vi "main.vi"() -> ()   [LabVIEW 2017]
uses:
  <vilib>/Instr/_visa.llb/VISA Configure Serial Port (Instr).vi
panel:
  in  "选项卡控件":enum32{"设置", "汽车状态", "电池状态", "单体电压", "单体温度"}(tab)
  in  "波特率":u32=19200
  in  "数据位":u16=8
  in  "奇偶位":enum16{"None", "Odd", "Even", "Mark", "Space"}(ring)
  in  "停止":bool
  in  "串口选择":refnum<visa-resource-name>="COM21"
  out "ID":string
  out "数据0":string
  out "数据1":string
  out "数据2":string
  out "数据3":string
  out "数据4":string
  out "数据5":string
  out "数据6":string
  out "数据7":string
  out "current time":timestamp
  out "error out":errorcluster
  out "轮速":u32(graph)
  out "单体温度断线告警":bool
  out "单体电压断线告警":bool
  out "充电状态":u8(ring) items=["停止充电", "进入充电", "恒流充电", "涓流充电", "充电完成"]
  out "车载充电器连接电阻":u8(ring) items=["InftyOmh", "220Omh", "680Omh", "未知电阻"]
  out "动力电池告警":bool
  out "动力电池告警级别":u32(ring) items=["无告警", "严重", "一般", "不严重"]
  out "动力电池总电压":dbl(graph)
  out "动力电池总电流":dbl(graph)
  out "剩余电量百分比":u32(graph)
  out "当前容量与出厂容量百分比":u32(graph)
  out "通信生命周期":u32(graph)
  out "动力电池状态":u32(ring) items=["无", "休眠", "自检", "待机", "预充", "正常运行", "关机", "故障"]
  out "最大允许充电功率":dbl
  out "最大允许充电电流":u16
  out "最大允许放电电流":u16
  out "最大允许放电功率":dbl
  out "加热控制":bool
  out "冷却控制":bool
  out "输出高压命令":bool
  out "关机命令":bool
  out "车载充电继电器开关":bool
  out "预充继电器开关":bool
  out "总负继电器开关":bool
  out "总正继电器开关":bool
  out "非车载充电继电器开关":bool
  out "非车载充电器连接确认":bool
  out "充电机在线":bool
  out "车载充电继电器错误":bool
  out "预充继电器错误":bool
  out "总负继电器错误":bool
  out "总正继电器错误":bool
  out "非车载充电继电器错误":bool
  out "车载充电器连接确认":bool
  out "充电请求电压":u16
  out "充电请求电流":u16
  out "电池低温告警级别":u8(ring) items=["无告警", "严重", "一般", "不严重"]
  out "电池低温告警":bool
  out "电池高温告警级别":u8(ring) items=["无告警", "严重", "一般", "不严重"]
  out "单体欠压告警":bool
  out "单体欠压告警级别":u8(ring) items=["无告警", "严重", "一般", "不严重"]
  out "单体过压告警":bool
  out "单体过压告警级别":u8(ring) items=["无告警", "严重", "一般", "不严重"]
  out "电池高温告警":bool
  out "稳态充电过流告警":bool
  out "电池组剩余电量百分比过低告警":bool caption="电池组剩余电量百分比过低告"
  out "电池组剩余电量百分比过高告警":bool
  out "整组欠压告警":bool
  out "被动均衡采集模块离线告警":bool
  out "整组过压告警":bool
  out "电池温差过大告警":bool
  out "电池压差过大告警":bool
  out "电池压差过大告警级别":u8(ring) items=["无告警", "严重", "一般", "不严重"]
  out "电池温差过大告警级别":u8(ring) items=["无告警", "严重", "一般", "不严重"]
  out "整组过压告警级别":u8(ring) items=["无告警", "严重", "一般", "不严重"]
  out "电池管理模块故障告警":bool
  out "继电器故障告警":bool
  out "预充失败告警":bool
  out "被动均衡采集模块均衡故障告警":bool
  out "霍尔断线告警":bool
  out "电池高压异常告警":bool
  out "漏电流超限告警级别":u8(ring) items=["无告警", "严重", "一般", "不严重"]
  out "漏电流超限告警":bool
  out "稳态放电过流告警级别":u8(ring) items=["无告警", "严重", "一般", "不严重"]
  out "稳态放电过流告警":bool
  out "整组欠压告警级别":u8(ring) items=["无告警", "严重", "一般", "不严重"]
  out "稳态充电过流告警级别":u8(ring) items=["无告警", "严重", "一般", "不严重"]
  out "瞬态充电过流告警":bool
  out "瞬态充电过流告警级别":u8(ring) items=["无告警", "严重", "一般", "不严重"]
  out "瞬态放电过流告警级别":u8(ring) items=["无告警", "严重", "一般", "不严重"]
  out "瞬态放电过流告警":bool
  out "电池组剩余电量百分比过低告警级别":u8(ring) items=["无告警", "严重", "一般", "不严重"]
  out "电池组剩余电量百分比过高告警级别":u8(ring) items=["无告警", "严重", "一般", "不严重"]
  out "整车控制模块通讯超时告警级别":u8(ring) items=["无告警", "严重", "一般", "不严重"]
  out "整车控制模块通讯超时告警":bool
  out "被动均衡采集模块离线告警级别":u8(ring) items=["无告警", "严重", "一般", "不严重"]
  in  "选项卡控件 2":T1(tab)
  out "最高单体电压":u16(graph)
  out "最低单体电压":u16(graph)
  out "最高单体电压序号":u32(graph)
  out "最低单体电压序号":u32(graph)
  out "单体电压2":u32(graph)
  out "单体电压5":u32(graph)
  out "单体电压6":u32(graph)
  out "单体电压7":u32(graph)
  out "单体电压0":u32(graph)
  out "单体电压1":u32(graph)
  out "单体电压3":u32(graph)
  out "单体电压4":u32(graph)
  out "单体电压10":u32(graph)
  out "单体电压13":u32(graph)
  out "单体电压14":u32(graph)
  out "单体电压15":u32(graph)
  out "单体电压8":u32(graph)
  out "单体电压9":u32(graph)
  out "单体电压11":u32(graph)
  out "单体电压12":u32(graph)
  out "单体电压21":u32(graph)
  out "单体电压18":u32(graph)
  out "单体电压23":u32(graph)
  out "单体电压17":u32(graph)
  out "单体电压20":u32(graph)
  out "单体电压22":u32(graph)
  out "单体电压16":u32(graph)
  out "单体电压19":u32(graph)
  out "单体电压30":u32(graph)
  out "单体电压28":u32(graph)
  out "单体电压25":u32(graph)
  out "单体电压31":u32(graph)
  out "单体电压26":u32(graph)
  out "单体电压29":u32(graph)
  out "单体电压24":u32(graph)
  out "单体电压27":u32(graph)
  out "单体电压38":u32(graph)
  out "单体电压36":u32(graph)
  out "单体电压33":u32(graph)
  out "单体电压39":u32(graph)
  out "单体电压34":u32(graph)
  out "单体电压37":u32(graph)
  out "单体电压32":u32(graph)
  out "单体电压35":u32(graph)
  out "单体电压46":u32(graph)
  out "单体电压44":u32(graph)
  out "单体电压41":u32(graph)
  out "单体电压47":u32(graph)
  out "单体电压42":u32(graph)
  out "单体电压45":u32(graph)
  out "单体电压40":u32(graph)
  out "单体电压43":u32(graph)
  in  "选项卡控件 3":T2(tab)
  out "最低温度序号":u32(graph)
  out "最低温度":u32(graph)
  out "最高温度":u32(graph)
  out "最高温度序号":u32(graph)
  out "单体温度0":u32(graph)
  out "单体温度1":u32(graph)
  out "单体温度2":u32(graph)
  out "单体温度3":u32(graph)
  out "单体温度4":u32(graph)
  out "单体温度6":u32(graph)
  out "单体温度7":u32(graph)
  out "单体温度5":u32(graph)
  out "单体温度8":u32(graph)
  out "单体温度9":u32(graph)
  out "单体温度10":u32(graph)
  out "单体温度11":u32(graph)
  out "单体温度12":u32(graph)
  out "单体温度14":u32(graph)
  out "单体温度15":u32(graph)
  out "单体温度13":u32(graph)
  out "单体温度16":u32(graph)
  out "单体温度17":u32(graph)
  out "单体温度18":u32(graph)
  out "单体温度19":u32(graph)
  out "单体温度20":u32(graph)
  out "单体温度22":u32(graph)
  out "单体温度23":u32(graph)
  out "单体温度21":u32(graph)
  out "单体温度29":u32(graph)
  out "单体温度31":u32(graph)
  out "单体温度30":u32(graph)
  out "单体温度28":u32(graph)
  out "单体温度27":u32(graph)
  out "单体温度26":u32(graph)
  out "单体温度25":u32(graph)
  out "单体温度24":u32(graph)
  out "单体温度32":u32(graph)
  out "单体温度33":u32(graph)
  out "单体温度34":u32(graph)
  out "单体温度35":u32(graph)
  out "单体温度36":u32(graph)
  out "单体温度38":u32(graph)
  out "单体温度39":u32(graph)
  out "单体温度37":u32(graph)
  out "单体温度40":u32(graph)
  out "单体温度41":u32(graph)
  out "单体温度42":u32(graph)
  out "单体温度43":u32(graph)
  out "单体温度44":u32(graph)
  out "单体温度46":u32(graph)
  out "单体温度47":u32(graph)
  out "单体温度45":u32(graph)
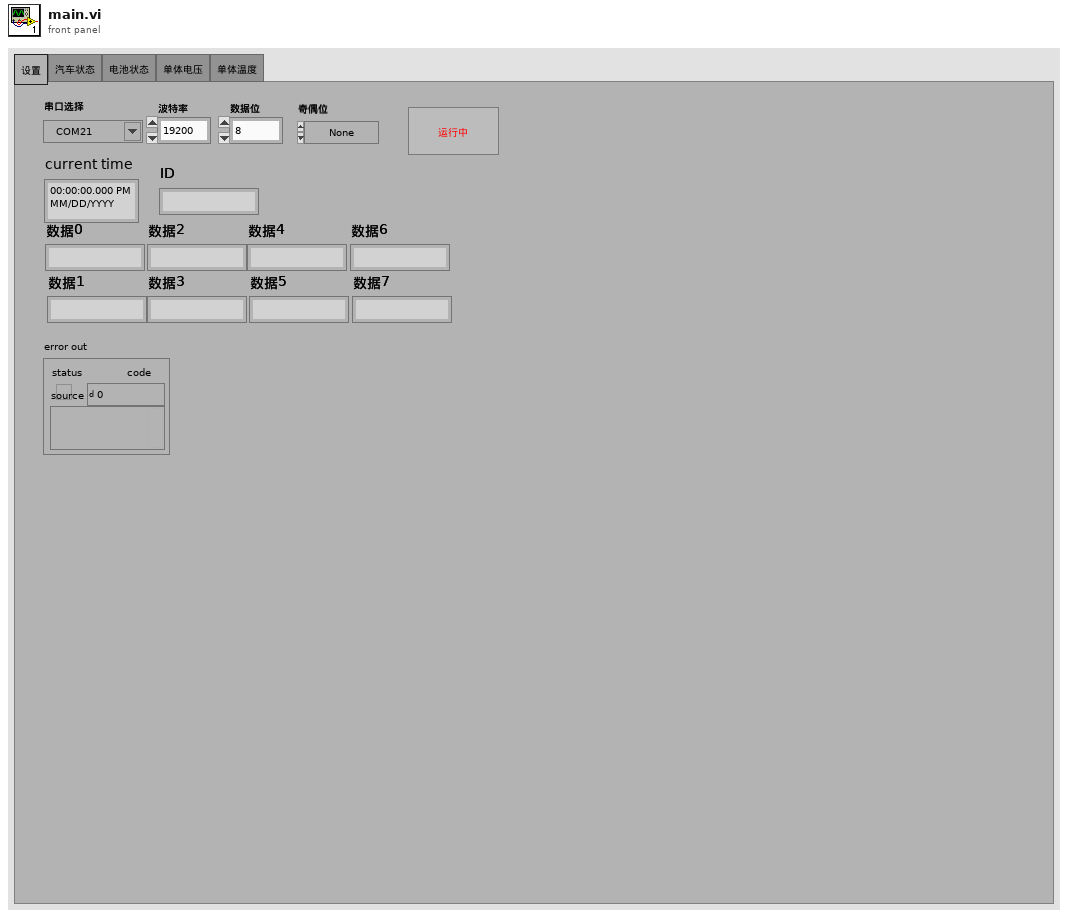
[diagram p1: front panel]
types:
  T1 = enum32{"危险单体电压", "单体电压0~7", "单体电压8~15", "单体电压16~23", "单体电压24~31", "单体电压32~39", "单体电压40~47"}
  T2 = enum32{"危险单体温度", "单体温度0~7", "单体温度8~15", "单体温度16~23", "单体温度24~31", "单体温度32~39", "单体温度40~47"}
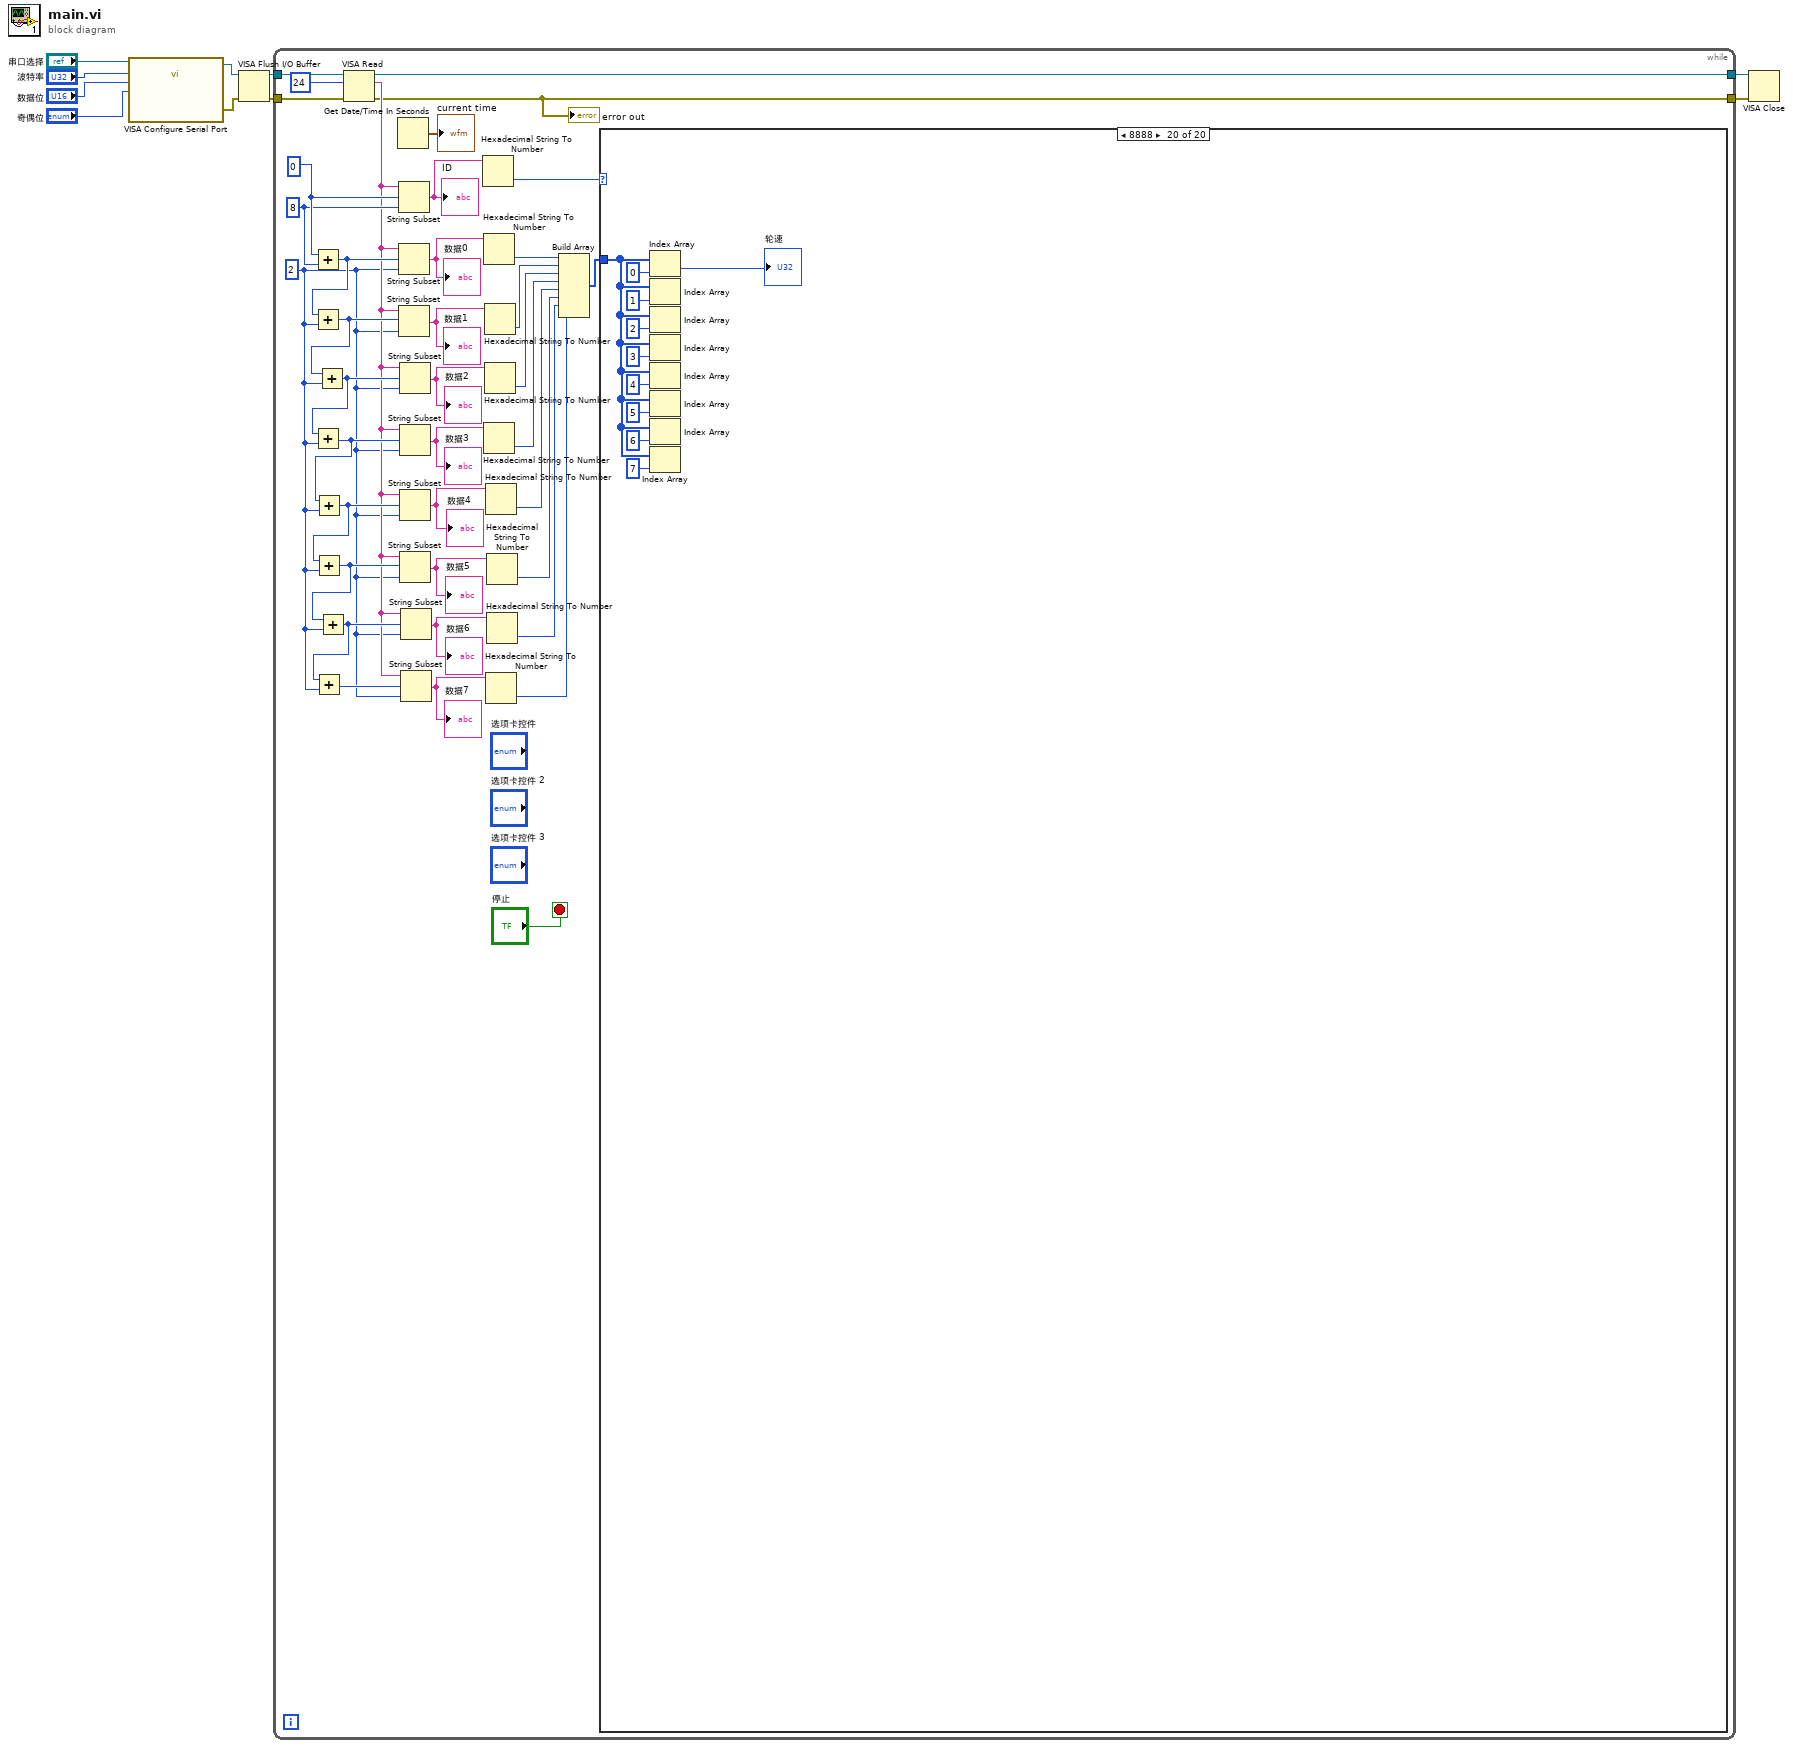
[diagram p0: block diagram]
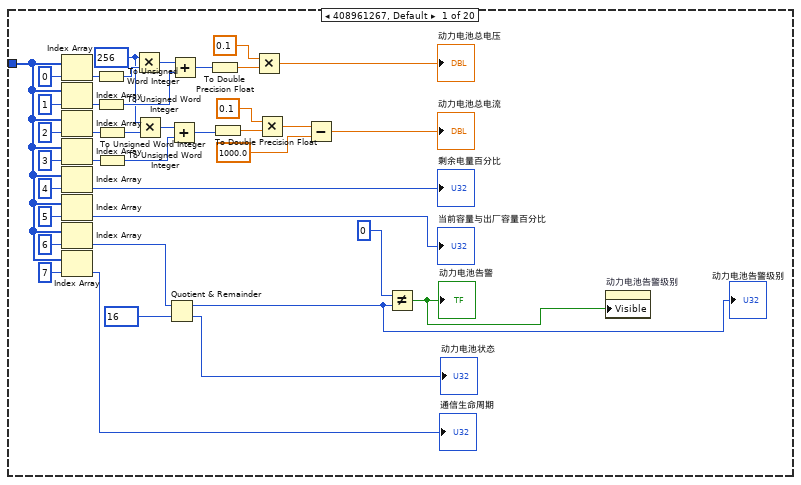
[diagram p2: hidden frame]
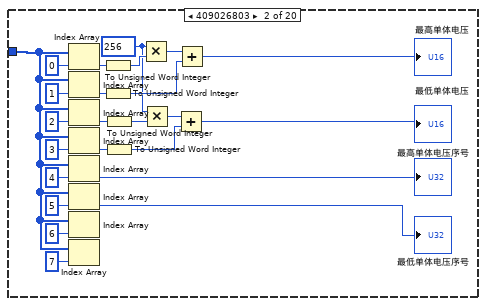
[diagram p3: hidden frame]
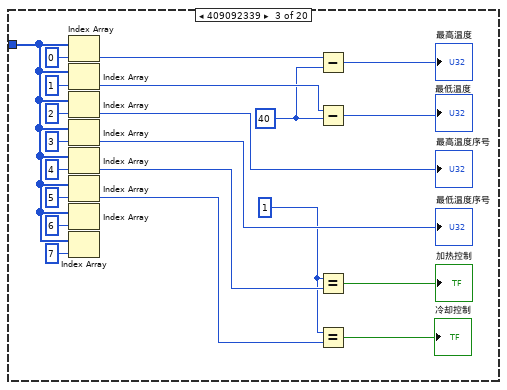
[diagram p4: hidden frame]
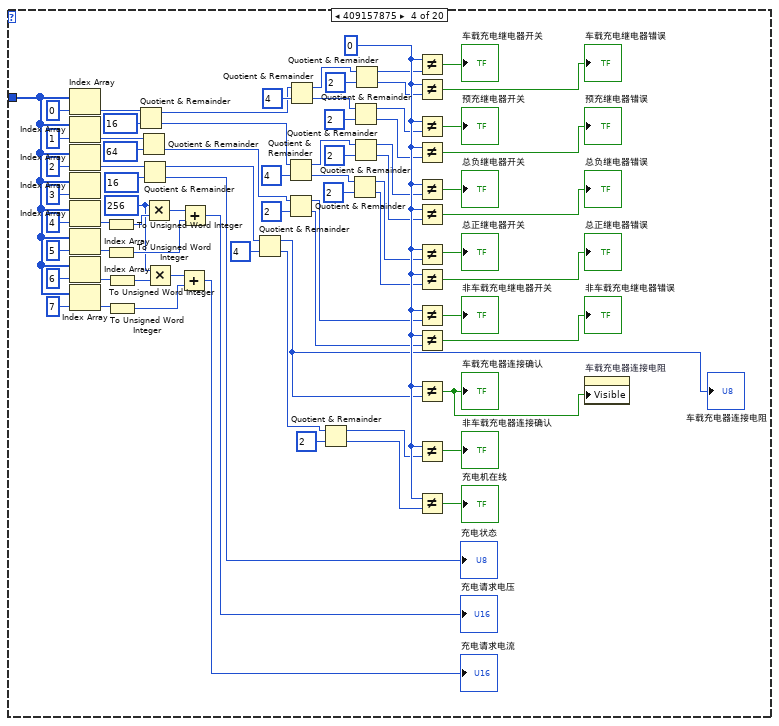
[diagram p5: hidden frame]
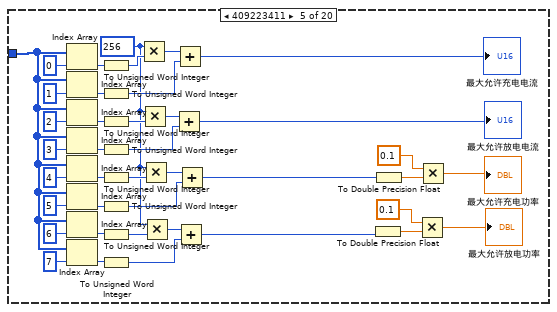
[diagram p6: hidden frame]
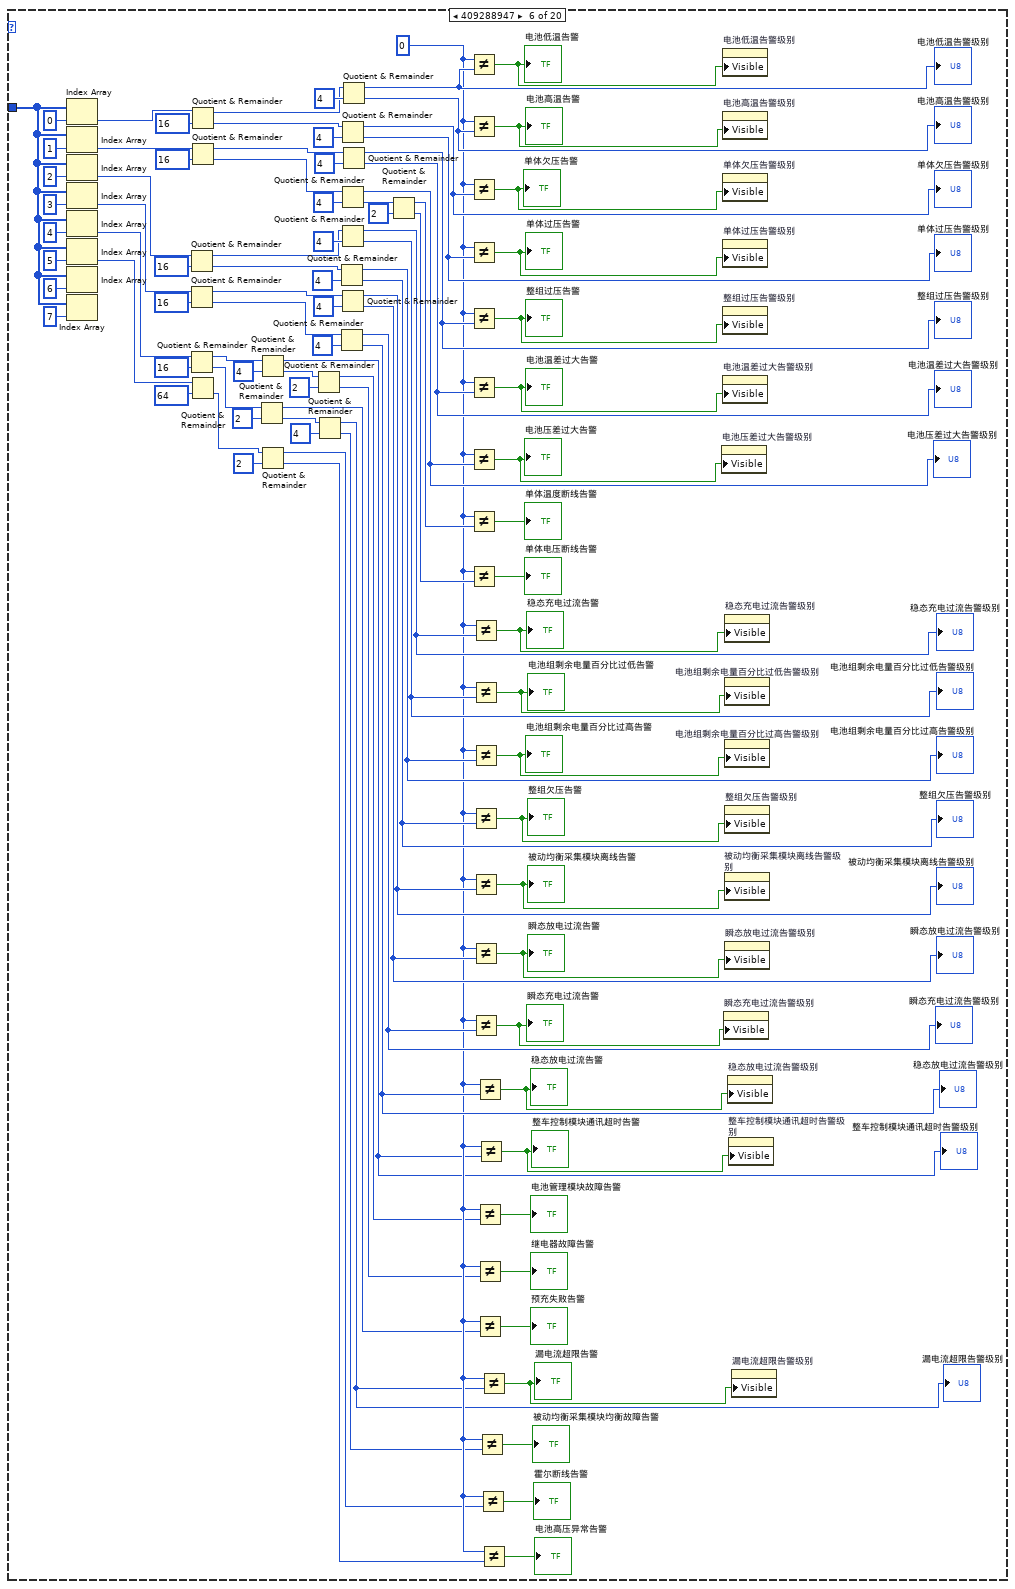
[diagram p7: hidden frame]
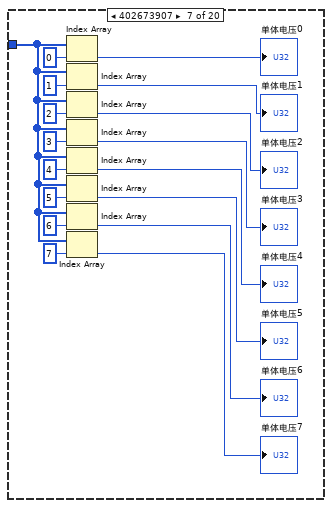
[diagram p8: hidden frame]
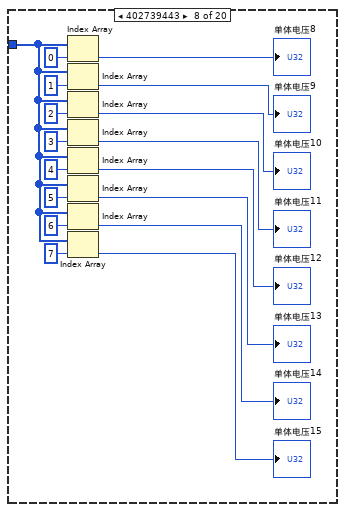
[diagram p9: hidden frame]
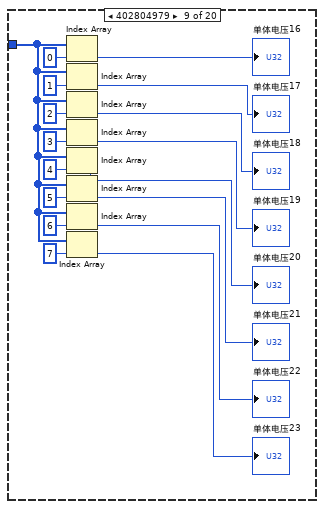
[diagram p10: hidden frame]
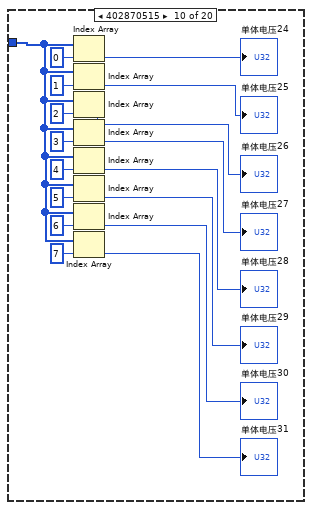
[diagram p11: hidden frame]
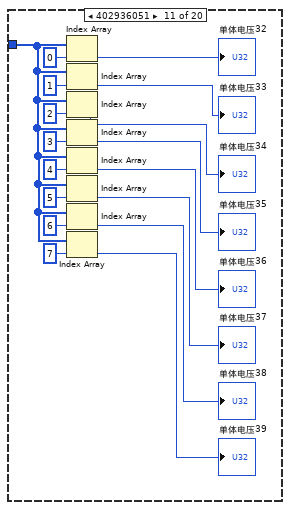
[diagram p12: hidden frame]
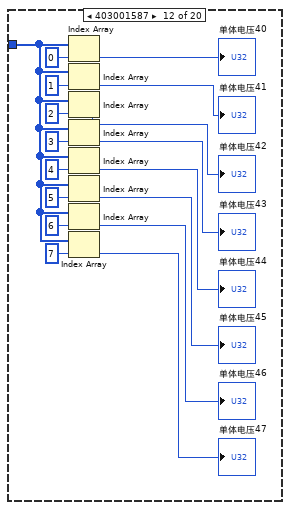
[diagram p13: hidden frame]
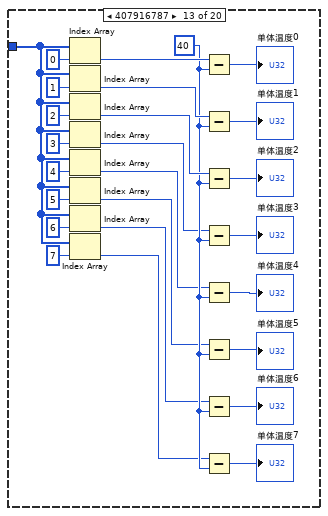
[diagram p14: hidden frame]
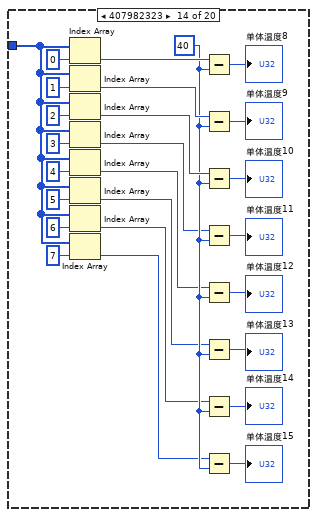
[diagram p15: hidden frame]
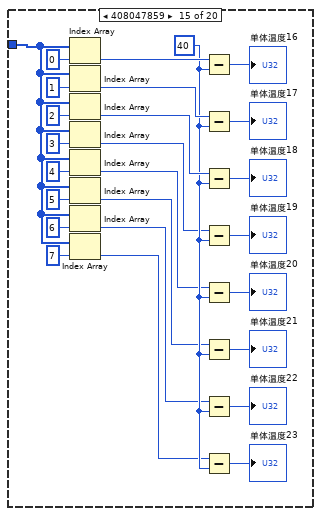
[diagram p16: hidden frame]
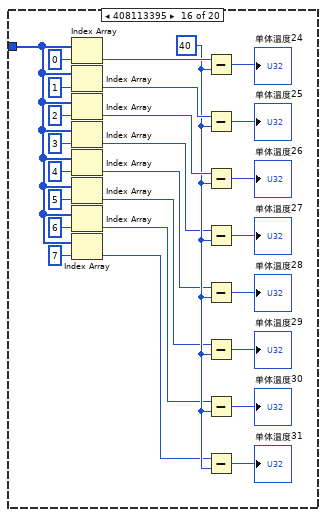
[diagram p17: hidden frame]
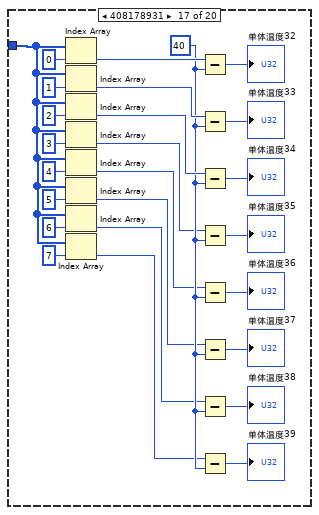
[diagram p18: hidden frame]
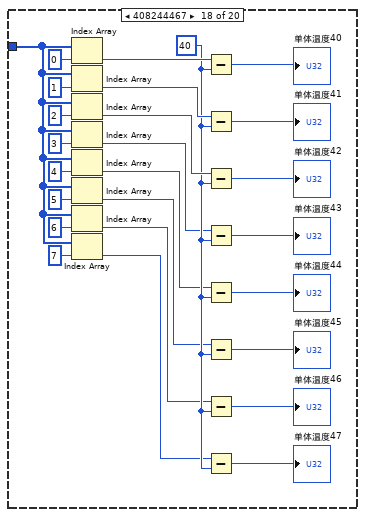
[diagram p19: hidden frame]
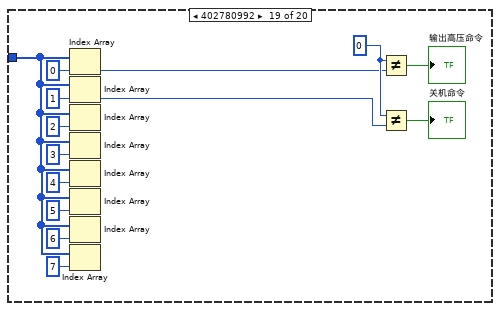
[diagram p20: hidden frame]
diagram:
  n1 = call-poly "VISA Configure Serial Port"("VISA resource name"="串口选择", "baud rate (9600)"="波特率", "data bits (8)"="数据位", "parity (0:none)"="奇偶位") -> ("VISA resource name out"=w10:refnum<visa-resource-name>, "error out"=w9:errorcluster)  [unwired: 10 in]
  n2 = VISA Flush I/O Buffer(VISA resource name=w10, error in (no error)=w9) -> (VISA resource name out=w5:refnum<visa-resource-name>, error out=w6:errorcluster)  [unwired: 1 in]
  n3 = while {
    tunnel: w6 -> [w47]
    tunnel: w5 -> [w46]
    tunnel: [w45] -> w4
    tunnel: [w11] -> w3
    stop <- "停止" stop-if-true
    w12 = u32 2 ("长度0")
    w33 = u32 8 ("长度0")
    w41 = u32 0 ("偏移0")
    n4 = Add(x=w41, y=w33) -> (x+y=w40:u32)
    n5 = Add(x=w40, y=w12) -> (x+y=w39:u32)
    n6 = Add(x=w39, y=w12) -> (x+y=w38:u32)
    n7 = Add(x=w38, y=w12) -> (x+y=w32:u32)
    n8 = Add(x=w32, y=w12) -> (x+y=w37:u32)
    n9 = Add(x=w37, y=w12) -> (x+y=w36:u32)
    n10 = Add(x=w36, y=w12) -> (x+y=w35:u32)
    n11 = Add(x=w35, y=w12) -> (x+y=w34:u32)
    n12 = VISA Read(VISA resource name=w46, byte count=u32 24, error in (no error)=w47) -> (VISA resource name out=w45:refnum<visa-resource-name>, read buffer=w15:string, error out=w11:errorcluster)  [unwired: 1 out]
    "error out" <- w11
    n13 = Get Date/Time In Seconds() -> (seconds since 1Jan1904=→"current time":timestamp)
    n14 = String Subset(string=w15, offset (0)=w41, length (rest)=w33) -> (substring=w43:string)
    "ID" <- w43
    n15 = String Subset(string=w15, offset (0)=w40, length (rest)=w12) -> (substring=w23:string)
    "数据0" <- w23
    n16 = String Subset(string=w15, offset (0)=w39, length (rest)=w12) -> (substring=w22:string)
    "数据1" <- w22
    n17 = String Subset(string=w15, offset (0)=w38, length (rest)=w12) -> (substring=w21:string)
    "数据2" <- w21
    n18 = String Subset(string=w15, offset (0)=w32, length (rest)=w12) -> (substring=w20:string)
    "数据3" <- w20
    n19 = String Subset(string=w15, offset (0)=w37, length (rest)=w12) -> (substring=w19:string)
    "数据4" <- w19
    n20 = String Subset(string=w15, offset (0)=w36, length (rest)=w12) -> (substring=w18:string)
    "数据5" <- w18
    n21 = String Subset(string=w15, offset (0)=w35, length (rest)=w12) -> (substring=w17:string)
    "数据6" <- w17
    n22 = String Subset(string=w15, offset (0)=w34, length (rest)=w12) -> (substring=w16:string)
    "数据7" <- w16
    n23 = Hexadecimal String To Number(string=w43) -> (number=w44:u32)  [unwired: 2 in, 1 out]
    n24 = Hexadecimal String To Number(string=w23) -> (number=w42:u32)  [unwired: 2 in, 1 out]
    n25 = Hexadecimal String To Number(string=w20) -> (number=w29:u32)  [unwired: 2 in, 1 out]
    n26 = Hexadecimal String To Number(string=w22) -> (number=w31:u32)  [unwired: 2 in, 1 out]
    n27 = Hexadecimal String To Number(string=w21) -> (number=w30:u32)  [unwired: 2 in, 1 out]
    n28 = Hexadecimal String To Number(string=w19) -> (number=w28:u32)  [unwired: 2 in, 1 out]
    n29 = Hexadecimal String To Number(string=w16) -> (number=w25:u32)  [unwired: 2 in, 1 out]
    n30 = Hexadecimal String To Number(string=w18) -> (number=w27:u32)  [unwired: 2 in, 1 out]
    n31 = Hexadecimal String To Number(string=w17) -> (number=w26:u32)  [unwired: 2 in, 1 out]
    n32 = Build Array(w42, w31, w30, w29, w28, w27, w26, w25) -> (w24:u32[])
    n33 = case shown="8888" w44 {
      tunnel: w24 -> [w79 w92 w124 w198 w228 w338 w355 w372 w389 w406 w423 w440 w466 w483 w509 w535 w561 w587 w610 w620]
      frame 408961267, Default {
        w68 = u16 256
        n34 = Index Array(array=w79, index=0) -> (element=w78:u32)
        n35 = Index Array(array=w79, index=1) -> (element=w75:u32)
        n36 = Index Array(array=w79, index=2) -> (element=w70:u32)
        n37 = Index Array(array=w79, index=3) -> (element=w69:u32)
        n38 = Index Array(array=w79, index=4) -> (element=→"剩余电量百分比":u32)
        n39 = Index Array(array=w79, index=5) -> (element=→"当前容量与出厂容量百分比":u32)
        n40 = Index Array(array=w79, index=6) -> (element=w63:u32)
        n41 = Index Array(array=w79, index=7) -> (element=→"通信生命周期":u32)
        n42 = To Unsigned Word Integer(number=w78) -> (unsigned 16bit integer=w77:u16)
        n43 = To Unsigned Word Integer(number=w75) -> (unsigned 16bit integer=w74:u16)
        n44 = To Unsigned Word Integer(number=w70) -> (unsigned 16bit integer=w73:u16)
        n45 = To Unsigned Word Integer(number=w69) -> (unsigned 16bit integer=w71:u16)
        n46 = Multiply(x=w68, y=w77) -> (x*y=w76:u16)
        n47 = Multiply(x=w68, y=w73) -> (x*y=w72:u16)
        n48 = Quotient & Remainder(x=w63, y=u32 16) -> (x-y*floor(x/y)=w49:u32, floor(x/y)=→"动力电池状态":u32)
        "动力电池告警级别" <- w49
        n49 = Add(x=w72, y=w71) -> (x+y=w54:u16)
        n50 = Add(x=w76, y=w74) -> (x+y=w60:u16)
        n51 = To Double Precision Float(number=w60) -> (double precision float=w57:dbl)
        n52 = To Double Precision Float(number=w54) -> (double precision float=w55:dbl)
        n53 = Multiply(x=0.1, y=w57) -> (x*y=→"动力电池总电压":dbl)
        n54 = Multiply(x=0.1, y=w55) -> (x*y=w53:dbl)
        n55 = Subtract(x=w53, y=1000.0) -> (x-y=→"动力电池总电流":dbl)
        n56 = Not Equal?(x=u32 0, y=w49) -> (x != y?=w50:bool)
        "动力电池告警" <- w50
        n57 = property on="动力电池告警级别" class="Ring (严格)"("Visible"=w50) -> ()  [unwired: 2 in, 2 out]
      }
      frame 409026803 {
        w93 = u16 256
        n58 = Index Array(array=w92, index=0) -> (element=w103:u32)
        n59 = Index Array(array=w92, index=1) -> (element=w100:u32)
        n60 = Index Array(array=w92, index=2) -> (element=w95:u32)
        n61 = Index Array(array=w92, index=3) -> (element=w94:u32)
        n62 = Index Array(array=w92, index=4) -> (element=→"最高单体电压序号":u32)
        n63 = Index Array(array=w92, index=5) -> (element=→"最低单体电压序号":u32)
        n64 = Index Array(array=w92, index=6) -> ()  [unwired: 1 out]
        n65 = Index Array(array=w92, index=7) -> ()  [unwired: 1 out]
        n66 = To Unsigned Word Integer(number=w103) -> (unsigned 16bit integer=w102:u16)
        n67 = To Unsigned Word Integer(number=w100) -> (unsigned 16bit integer=w99:u16)
        n68 = To Unsigned Word Integer(number=w95) -> (unsigned 16bit integer=w98:u16)
        n69 = To Unsigned Word Integer(number=w94) -> (unsigned 16bit integer=w96:u16)
        n70 = Multiply(x=w93, y=w102) -> (x*y=w101:u16)
        n71 = Multiply(x=w93, y=w98) -> (x*y=w97:u16)
        n72 = Add(x=w97, y=w96) -> (x+y=→"最低单体电压":u16)
        n73 = Add(x=w101, y=w99) -> (x+y=→"最高单体电压":u16)
      }
      frame 409092339 {
        w112 = u8 1
        w119 = u8 40
        n74 = Index Array(array=w124, index=0) -> (element=w122:u32)
        n75 = Index Array(array=w124, index=1) -> (element=w120:u32)
        n76 = Index Array(array=w124, index=2) -> (element=→"最高温度序号":u32)
        n77 = Index Array(array=w124, index=3) -> (element=→"最低温度序号":u32)
        n78 = Index Array(array=w124, index=4) -> (element=w114:u32)
        n79 = Index Array(array=w124, index=5) -> (element=w113:u32)
        n80 = Index Array(array=w124, index=6) -> ()  [unwired: 1 out]
        n81 = Index Array(array=w124, index=7) -> ()  [unwired: 1 out]
        n82 = Subtract(x=w122, y=w119) -> (x-y=→"最高温度":u32)
        n83 = Subtract(x=w120, y=w119) -> (x-y=→"最低温度":u32)
        n84 = Equal?(x=w112, y=w114) -> (x = y?=→"加热控制":bool)
        n85 = Equal?(x=w112, y=w113) -> (x = y?=→"冷却控制":bool)
      }
      frame 409157875 {
        w139 = u16 256
        w179 = u8 0
        n86 = Index Array(array=w198, index=0) -> (element=w196:u32)
        n87 = Index Array(array=w198, index=1) -> (element=w182:u32)
        n88 = Index Array(array=w198, index=2) -> (element=w155:u32)
        n89 = Index Array(array=w198, index=3) -> ()  [unwired: 1 out]
        n90 = Index Array(array=w198, index=4) -> (element=w138:u32)
        n91 = Index Array(array=w198, index=5) -> (element=w137:u32)
        n92 = Index Array(array=w198, index=6) -> (element=w136:u32)
        n93 = Index Array(array=w198, index=7) -> (element=w135:u32)
        n94 = To Unsigned Word Integer(number=w138) -> (unsigned 16bit integer=w145:u16)
        n95 = To Unsigned Word Integer(number=w137) -> (unsigned 16bit integer=w143:u16)
        n96 = To Unsigned Word Integer(number=w136) -> (unsigned 16bit integer=w142:u16)
        n97 = To Unsigned Word Integer(number=w135) -> (unsigned 16bit integer=w140:u16)
        n98 = Quotient & Remainder(x=w196, y=u8 16) -> (x-y*floor(x/y)=w193:u32, floor(x/y)=w192:u32)
        n99 = Quotient & Remainder(x=w182, y=u8 64) -> (floor(x/y)=w159:u32)  [unwired: 1 out]
        n100 = Quotient & Remainder(x=w155, y=u8 16) -> (x-y*floor(x/y)=w153:u32, floor(x/y)=→"充电状态":u32)
        n101 = Multiply(x=w139, y=w145) -> (x*y=w144:u16)
        n102 = Multiply(x=w139, y=w142) -> (x*y=w141:u16)
        n103 = Add(x=w141, y=w140) -> (x+y=→"充电请求电流":u16)
        n104 = Add(x=w144, y=w143) -> (x+y=→"充电请求电压":u16)
        n105 = Quotient & Remainder(x=w153, y=u8 4) -> (x-y*floor(x/y)=w148:u32, floor(x/y)=w151:u32)
        "车载充电器连接电阻" <- w148
        n106 = Quotient & Remainder(x=w192, y=u8 4) -> (x-y*floor(x/y)=w185:u32, floor(x/y)=w184:u32)
        n107 = Quotient & Remainder(x=w159, y=u8 2) -> (x-y*floor(x/y)=w158:u32, floor(x/y)=w157:u32)
        n108 = Quotient & Remainder(x=w193, y=u8 4) -> (x-y*floor(x/y)=w187:u32, floor(x/y)=w186:u32)
        n109 = Quotient & Remainder(x=w151, y=u8 2) -> (x-y*floor(x/y)=w149:u32, floor(x/y)=w150:u32)
        n110 = Quotient & Remainder(x=w184, y=u8 2) -> (x-y*floor(x/y)=w166:u32, floor(x/y)=w167:u32)
        n111 = Quotient & Remainder(x=w186, y=u8 2) -> (x-y*floor(x/y)=w162:u32, floor(x/y)=w163:u32)
        n112 = Quotient & Remainder(x=w185, y=u8 2) -> (x-y*floor(x/y)=w164:u32, floor(x/y)=w165:u32)
        n113 = Quotient & Remainder(x=w187, y=u8 2) -> (x-y*floor(x/y)=w168:u32, floor(x/y)=w161:u32)
        n114 = Not Equal?(x=w179, y=w168) -> (x != y?=→"车载充电继电器开关":bool)
        n115 = Not Equal?(x=w179, y=w161) -> (x != y?=→"车载充电继电器错误":bool)
        n116 = Not Equal?(x=w179, y=w162) -> (x != y?=→"预充继电器开关":bool)
        n117 = Not Equal?(x=w179, y=w163) -> (x != y?=→"预充继电器错误":bool)
        n118 = Not Equal?(x=w179, y=w164) -> (x != y?=→"总负继电器开关":bool)
        n119 = Not Equal?(x=w179, y=w165) -> (x != y?=→"总负继电器错误":bool)
        n120 = Not Equal?(x=w179, y=w166) -> (x != y?=→"总正继电器开关":bool)
        n121 = Not Equal?(x=w179, y=w167) -> (x != y?=→"总正继电器错误":bool)
        n122 = Not Equal?(x=w179, y=w158) -> (x != y?=→"非车载充电继电器开关":bool)
        n123 = Not Equal?(x=w179, y=w157) -> (x != y?=→"非车载充电继电器错误":bool)
        n124 = Not Equal?(x=w179, y=w148) -> (x != y?=w147:bool)
        "车载充电器连接确认" <- w147
        n125 = Not Equal?(x=w179, y=w149) -> (x != y?=→"非车载充电器连接确认":bool)
        n126 = Not Equal?(x=w179, y=w150) -> (x != y?=→"充电机在线":bool)
        n127 = property on="车载充电器连接电阻" class="Ring (严格)"("Visible"=w147) -> ()  [unwired: 2 in, 2 out]
      }
      frame 409223411 {
        w217 = u16 256
        n128 = Index Array(array=w228, index=0) -> (element=w237:u32)
        n129 = Index Array(array=w228, index=1) -> (element=w240:u32)
        n130 = Index Array(array=w228, index=2) -> (element=w245:u32)
        n131 = Index Array(array=w228, index=3) -> (element=w246:u32)
        n132 = Index Array(array=w228, index=4) -> (element=w216:u32)
        n133 = Index Array(array=w228, index=5) -> (element=w215:u32)
        n134 = Index Array(array=w228, index=6) -> (element=w214:u32)
        n135 = Index Array(array=w228, index=7) -> (element=w213:u32)
        n136 = To Unsigned Word Integer(number=w237) -> (unsigned 16bit integer=w238:u16)
        n137 = To Unsigned Word Integer(number=w240) -> (unsigned 16bit integer=w241:u16)
        n138 = To Unsigned Word Integer(number=w245) -> (unsigned 16bit integer=w242:u16)
        n139 = To Unsigned Word Integer(number=w246) -> (unsigned 16bit integer=w244:u16)
        n140 = To Unsigned Word Integer(number=w216) -> (unsigned 16bit integer=w218:u16)
        n141 = To Unsigned Word Integer(number=w215) -> (unsigned 16bit integer=w220:u16)
        n142 = To Unsigned Word Integer(number=w214) -> (unsigned 16bit integer=w221:u16)
        n143 = To Unsigned Word Integer(number=w213) -> (unsigned 16bit integer=w223:u16)
        n144 = Multiply(x=w217, y=w238) -> (x*y=w239:u16)
        n145 = Multiply(x=w217, y=w242) -> (x*y=w243:u16)
        n146 = Multiply(x=w217, y=w218) -> (x*y=w219:u16)
        n147 = Multiply(x=w217, y=w221) -> (x*y=w222:u16)
        n148 = Add(x=w243, y=w244) -> (x+y=→"最大允许放电电流":u16)
        n149 = Add(x=w239, y=w241) -> (x+y=→"最大允许充电电流":u16)
        n150 = Add(x=w222, y=w223) -> (x+y=w211:u16)
        n151 = Add(x=w219, y=w220) -> (x+y=w212:u16)
        n152 = To Double Precision Float(number=w211) -> (double precision float=w224:dbl)
        n153 = To Double Precision Float(number=w212) -> (double precision float=w226:dbl)
        n154 = Multiply(x=0.1, y=w224) -> (x*y=→"最大允许放电功率":dbl)
        n155 = Multiply(x=0.1, y=w226) -> (x*y=→"最大允许充电功率":dbl)
      }
      frame 409288947 {
        w266 = u8 0
        n156 = Index Array(array=w338, index=0) -> (element=w329:u32)
        n157 = Index Array(array=w338, index=1) -> (element=w320:u32)
        n158 = Index Array(array=w338, index=2) -> (element=w292:u32)
        n159 = Index Array(array=w338, index=3) -> (element=w291:u32)
        n160 = Index Array(array=w338, index=4) -> (element=w260:u32)
        n161 = Index Array(array=w338, index=5) -> (element=w249:u32)
        n162 = Index Array(array=w338, index=6) -> ()  [unwired: 1 out]
        n163 = Index Array(array=w338, index=7) -> ()  [unwired: 1 out]
        n164 = Quotient & Remainder(x=w292, y=u8 16) -> (x-y*floor(x/y)=w299:u32, floor(x/y)=w298:u32)
        n165 = Quotient & Remainder(x=w291, y=u8 16) -> (x-y*floor(x/y)=w294:u32, floor(x/y)=w293:u32)
        n166 = Quotient & Remainder(x=w260, y=u8 16) -> (x-y*floor(x/y)=w262:u32, floor(x/y)=w261:u32)
        n167 = Quotient & Remainder(x=w329, y=u8 16) -> (x-y*floor(x/y)=w334:u32, floor(x/y)=w333:u32)
        n168 = Quotient & Remainder(x=w320, y=u8 16) -> (x-y*floor(x/y)=w322:u32, floor(x/y)=w321:u32)
        n169 = Quotient & Remainder(x=w249, y=u8 64) -> (floor(x/y)=w330:u32)  [unwired: 1 out]
        n170 = Quotient & Remainder(x=w261, y=u8 2) -> (x-y*floor(x/y)=w252:u32, floor(x/y)=w254:u32)
        n171 = Quotient & Remainder(x=w262, y=u8 4) -> (x-y*floor(x/y)=w259:u32, floor(x/y)=w257:u32)
        "整车控制模块通讯超时告警级别" <- w259
        n172 = Quotient & Remainder(x=w330, y=u8 2) -> (x-y*floor(x/y)=w247:u32, floor(x/y)=w248:u32)
        n173 = Quotient & Remainder(x=w257, y=u8 2) -> (x-y*floor(x/y)=w256:u32, floor(x/y)=w253:u32)
        n174 = Quotient & Remainder(x=w254, y=u8 4) -> (x-y*floor(x/y)=w250:u32, floor(x/y)=w251:u32)
        "漏电流超限告警级别" <- w250
        n175 = Quotient & Remainder(x=w298, y=u8 4) -> (x-y*floor(x/y)=w282:u32, floor(x/y)=w281:u32)
        "电池组剩余电量百分比过高告警级别" <- w282
        "整组欠压告警级别" <- w281
        n176 = Quotient & Remainder(x=w293, y=u8 4) -> (x-y*floor(x/y)=w278:u32, floor(x/y)=w277:u32)
        "瞬态充电过流告警级别" <- w278
        "稳态放电过流告警级别" <- w277
        n177 = Quotient & Remainder(x=w333, y=u8 4) -> (x-y*floor(x/y)=w314:u32, floor(x/y)=w313:u32)
        "单体欠压告警级别" <- w314
        "单体过压告警级别" <- w313
        n178 = Quotient & Remainder(x=w321, y=u8 4) -> (x-y*floor(x/y)=w308:u32, floor(x/y)=w307:u32)
        "电池压差过大告警级别" <- w308
        n179 = Quotient & Remainder(x=w299, y=u8 4) -> (x-y*floor(x/y)=w284:u32, floor(x/y)=w283:u32)
        "稳态充电过流告警级别" <- w284
        "电池组剩余电量百分比过低告警级别" <- w283
        n180 = Quotient & Remainder(x=w294, y=u8 4) -> (x-y*floor(x/y)=w280:u32, floor(x/y)=w279:u32)
        "被动均衡采集模块离线告警级别" <- w280
        "瞬态放电过流告警级别" <- w279
        n181 = Quotient & Remainder(x=w334, y=u8 4) -> (x-y*floor(x/y)=w328:u32, floor(x/y)=w326:u32)
        "电池低温告警级别" <- w328
        "电池高温告警级别" <- w326
        n182 = Quotient & Remainder(x=w322, y=u8 4) -> (x-y*floor(x/y)=w312:u32, floor(x/y)=w309:u32)
        "整组过压告警级别" <- w312
        "电池温差过大告警级别" <- w309
        n183 = Quotient & Remainder(x=w307, y=u8 2) -> (x-y*floor(x/y)=w304:u32, floor(x/y)=w303:u32)
        n184 = Not Equal?(x=w266, y=w328) -> (x != y?=w327:bool)
        "电池低温告警" <- w327
        n185 = Not Equal?(x=w266, y=w326) -> (x != y?=w318:bool)
        "电池高温告警" <- w318
        n186 = Not Equal?(x=w266, y=w314) -> (x != y?=w317:bool)
        "单体欠压告警" <- w317
        n187 = Not Equal?(x=w266, y=w313) -> (x != y?=w316:bool)
        "单体过压告警" <- w316
        n188 = Not Equal?(x=w266, y=w312) -> (x != y?=w315:bool)
        "整组过压告警" <- w315
        n189 = Not Equal?(x=w266, y=w309) -> (x != y?=w311:bool)
        "电池温差过大告警" <- w311
        n190 = Not Equal?(x=w266, y=w308) -> (x != y?=w310:bool)
        "电池压差过大告警" <- w310
        n191 = Not Equal?(x=w266, y=w304) -> (x != y?=→"单体温度断线告警":bool)
        n192 = Not Equal?(x=w266, y=w303) -> (x != y?=→"单体电压断线告警":bool)
        n193 = Not Equal?(x=w266, y=w284) -> (x != y?=w290:bool)
        "稳态充电过流告警" <- w290
        n194 = Not Equal?(x=w266, y=w283) -> (x != y?=w289:bool)
        "电池组剩余电量百分比过低告警" <- w289
        n195 = Not Equal?(x=w266, y=w282) -> (x != y?=w288:bool)
        "电池组剩余电量百分比过高告警" <- w288
        n196 = Not Equal?(x=w266, y=w281) -> (x != y?=w287:bool)
        "整组欠压告警" <- w287
        n197 = Not Equal?(x=w266, y=w280) -> (x != y?=w286:bool)
        "被动均衡采集模块离线告警" <- w286
        n198 = Not Equal?(x=w266, y=w279) -> (x != y?=w285:bool)
        "瞬态放电过流告警" <- w285
        n199 = Not Equal?(x=w266, y=w278) -> (x != y?=w275:bool)
        "瞬态充电过流告警" <- w275
        n200 = Not Equal?(x=w266, y=w277) -> (x != y?=w276:bool)
        "稳态放电过流告警" <- w276
        n201 = Not Equal?(x=w266, y=w256) -> (x != y?=→"电池管理模块故障告警":bool)
        n202 = Not Equal?(x=w266, y=w253) -> (x != y?=→"继电器故障告警":bool)
        n203 = Not Equal?(x=w266, y=w252) -> (x != y?=→"预充失败告警":bool)
        n204 = Not Equal?(x=w266, y=w259) -> (x != y?=w272:bool)
        "整车控制模块通讯超时告警" <- w272
        n205 = Not Equal?(x=w266, y=w251) -> (x != y?=→"被动均衡采集模块均衡故障告警":bool)
        n206 = Not Equal?(x=w266, y=w247) -> (x != y?=→"霍尔断线告警":bool)
        n207 = Not Equal?(x=w266, y=w250) -> (x != y?=w269:bool)
        "漏电流超限告警" <- w269
        n208 = Not Equal?(x=w266, y=w248) -> (x != y?=→"电池高压异常告警":bool)
        n209 = property on="电池压差过大告警级别" class="Ring (严格)"("Visible"=w310) -> ()  [unwired: 2 in, 2 out]
        n210 = property on="电池低温告警级别" class="Ring (严格)"("Visible"=w327) -> ()  [unwired: 2 in, 2 out]
        n211 = property on="电池高温告警级别" class="Ring (严格)"("Visible"=w318) -> ()  [unwired: 2 in, 2 out]
        n212 = property on="单体欠压告警级别" class="Ring (严格)"("Visible"=w317) -> ()  [unwired: 2 in, 2 out]
        n213 = property on="单体过压告警级别" class="Ring (严格)"("Visible"=w316) -> ()  [unwired: 2 in, 2 out]
        n214 = property on="整组过压告警级别" class="Ring (严格)"("Visible"=w315) -> ()  [unwired: 2 in, 2 out]
        n215 = property on="电池温差过大告警级别" class="Ring (严格)"("Visible"=w311) -> ()  [unwired: 2 in, 2 out]
        n216 = property on="瞬态充电过流告警级别" class="Ring (严格)"("Visible"=w275) -> ()  [unwired: 2 in, 2 out]
        n217 = property on="稳态充电过流告警级别" class="Ring (严格)"("Visible"=w290) -> ()  [unwired: 2 in, 2 out]
        n218 = property on="电池组剩余电量百分比过低告警级别" class="Ring (严格)"("Visible"=w289) -> ()  [unwired: 2 in, 2 out]
        n219 = property on="电池组剩余电量百分比过高告警级别" class="Ring (严格)"("Visible"=w288) -> ()  [unwired: 2 in, 2 out]
        n220 = property on="整组欠压告警级别" class="Ring (严格)"("Visible"=w287) -> ()  [unwired: 2 in, 2 out]
        n221 = property on="被动均衡采集模块离线告警级别" class="Ring (严格)"("Visible"=w286) -> ()  [unwired: 2 in, 2 out]
        n222 = property on="瞬态放电过流告警级别" class="Ring (严格)"("Visible"=w285) -> ()  [unwired: 2 in, 2 out]
        n223 = property on="稳态放电过流告警级别" class="Ring (严格)"("Visible"=w276) -> ()  [unwired: 2 in, 2 out]
        n224 = property on="整车控制模块通讯超时告警级别" class="Ring (严格)"("Visible"=w272) -> ()  [unwired: 2 in, 2 out]
        n225 = property on="漏电流超限告警级别" class="Ring (严格)"("Visible"=w269) -> ()  [unwired: 2 in, 2 out]
      }
      frame 402673907 {
        n226 = Index Array(array=w355, index=0) -> (element=→"单体电压0":u32)
        n227 = Index Array(array=w355, index=1) -> (element=→"单体电压1":u32)
        n228 = Index Array(array=w355, index=2) -> (element=→"单体电压2":u32)
        n229 = Index Array(array=w355, index=3) -> (element=→"单体电压3":u32)
        n230 = Index Array(array=w355, index=4) -> (element=→"单体电压4":u32)
        n231 = Index Array(array=w355, index=5) -> (element=→"单体电压5":u32)
        n232 = Index Array(array=w355, index=6) -> (element=→"单体电压6":u32)
        n233 = Index Array(array=w355, index=7) -> (element=→"单体电压7":u32)
      }
      frame 402739443 {
        n234 = Index Array(array=w372, index=0) -> (element=→"单体电压8":u32)
        n235 = Index Array(array=w372, index=1) -> (element=→"单体电压9":u32)
        n236 = Index Array(array=w372, index=2) -> (element=→"单体电压10":u32)
        n237 = Index Array(array=w372, index=3) -> (element=→"单体电压11":u32)
        n238 = Index Array(array=w372, index=4) -> (element=→"单体电压12":u32)
        n239 = Index Array(array=w372, index=5) -> (element=→"单体电压13":u32)
        n240 = Index Array(array=w372, index=6) -> (element=→"单体电压14":u32)
        n241 = Index Array(array=w372, index=7) -> (element=→"单体电压15":u32)
      }
      frame 402804979 {
        n242 = Index Array(array=w389, index=0) -> (element=→"单体电压16":u32)
        n243 = Index Array(array=w389, index=1) -> (element=→"单体电压17":u32)
        n244 = Index Array(array=w389, index=2) -> (element=→"单体电压18":u32)
        n245 = Index Array(array=w389, index=3) -> (element=→"单体电压19":u32)
        n246 = Index Array(array=w389, index=4) -> (element=→"单体电压20":u32)
        n247 = Index Array(array=w389, index=5) -> (element=→"单体电压21":u32)
        n248 = Index Array(array=w389, index=6) -> (element=→"单体电压22":u32)
        n249 = Index Array(array=w389, index=7) -> (element=→"单体电压23":u32)
      }
      frame 402870515 {
        n250 = Index Array(array=w406, index=0) -> (element=→"单体电压24":u32)
        n251 = Index Array(array=w406, index=1) -> (element=→"单体电压25":u32)
        n252 = Index Array(array=w406, index=2) -> (element=→"单体电压26":u32)
        n253 = Index Array(array=w406, index=3) -> (element=→"单体电压27":u32)
        n254 = Index Array(array=w406, index=4) -> (element=→"单体电压28":u32)
        n255 = Index Array(array=w406, index=5) -> (element=→"单体电压29":u32)
        n256 = Index Array(array=w406, index=6) -> (element=→"单体电压30":u32)
        n257 = Index Array(array=w406, index=7) -> (element=→"单体电压31":u32)
      }
      frame 402936051 {
        n258 = Index Array(array=w423, index=0) -> (element=→"单体电压32":u32)
        n259 = Index Array(array=w423, index=1) -> (element=→"单体电压33":u32)
        n260 = Index Array(array=w423, index=2) -> (element=→"单体电压34":u32)
        n261 = Index Array(array=w423, index=3) -> (element=→"单体电压35":u32)
        n262 = Index Array(array=w423, index=4) -> (element=→"单体电压36":u32)
        n263 = Index Array(array=w423, index=5) -> (element=→"单体电压37":u32)
        n264 = Index Array(array=w423, index=6) -> (element=→"单体电压38":u32)
        n265 = Index Array(array=w423, index=7) -> (element=→"单体电压39":u32)
      }
      frame 403001587 {
        n266 = Index Array(array=w440, index=0) -> (element=→"单体电压40":u32)
        n267 = Index Array(array=w440, index=1) -> (element=→"单体电压41":u32)
        n268 = Index Array(array=w440, index=2) -> (element=→"单体电压42":u32)
        n269 = Index Array(array=w440, index=3) -> (element=→"单体电压43":u32)
        n270 = Index Array(array=w440, index=4) -> (element=→"单体电压44":u32)
        n271 = Index Array(array=w440, index=5) -> (element=→"单体电压45":u32)
        n272 = Index Array(array=w440, index=6) -> (element=→"单体电压46":u32)
        n273 = Index Array(array=w440, index=7) -> (element=→"单体电压47":u32)
      }
      frame 407916787 {
        w459 = u8 40
        n274 = Index Array(array=w466, index=0) -> (element=w464:u32)
        n275 = Index Array(array=w466, index=1) -> (element=w462:u32)
        n276 = Index Array(array=w466, index=2) -> (element=w460:u32)
        n277 = Index Array(array=w466, index=3) -> (element=w449:u32)
        n278 = Index Array(array=w466, index=4) -> (element=w450:u32)
        n279 = Index Array(array=w466, index=5) -> (element=w451:u32)
        n280 = Index Array(array=w466, index=6) -> (element=w452:u32)
        n281 = Index Array(array=w466, index=7) -> (element=w453:u32)
        n282 = Subtract(x=w464, y=w459) -> (x-y=→"单体温度0":u32)
        n283 = Subtract(x=w462, y=w459) -> (x-y=→"单体温度1":u32)
        n284 = Subtract(x=w460, y=w459) -> (x-y=→"单体温度2":u32)
        n285 = Subtract(x=w449, y=w459) -> (x-y=→"单体温度3":u32)
        n286 = Subtract(x=w450, y=w459) -> (x-y=→"单体温度4":u32)
        n287 = Subtract(x=w451, y=w459) -> (x-y=→"单体温度5":u32)
        n288 = Subtract(x=w452, y=w459) -> (x-y=→"单体温度6":u32)
        n289 = Subtract(x=w453, y=w459) -> (x-y=→"单体温度7":u32)
      }
      frame 407982323 {
        w489 = u8 40
        n290 = Index Array(array=w483, index=0) -> (element=w492:u32)
        n291 = Index Array(array=w483, index=1) -> (element=w491:u32)
        n292 = Index Array(array=w483, index=2) -> (element=w490:u32)
        n293 = Index Array(array=w483, index=3) -> (element=w484:u32)
        n294 = Index Array(array=w483, index=4) -> (element=w485:u32)
        n295 = Index Array(array=w483, index=5) -> (element=w486:u32)
        n296 = Index Array(array=w483, index=6) -> (element=w487:u32)
        n297 = Index Array(array=w483, index=7) -> (element=w488:u32)
        n298 = Subtract(x=w492, y=w489) -> (x-y=→"单体温度8":u32)
        n299 = Subtract(x=w491, y=w489) -> (x-y=→"单体温度9":u32)
        n300 = Subtract(x=w490, y=w489) -> (x-y=→"单体温度10":u32)
        n301 = Subtract(x=w484, y=w489) -> (x-y=→"单体温度11":u32)
        n302 = Subtract(x=w485, y=w489) -> (x-y=→"单体温度12":u32)
        n303 = Subtract(x=w486, y=w489) -> (x-y=→"单体温度13":u32)
        n304 = Subtract(x=w487, y=w489) -> (x-y=→"单体温度14":u32)
        n305 = Subtract(x=w488, y=w489) -> (x-y=→"单体温度15":u32)
      }
      frame 408047859 {
        w515 = u8 40
        n306 = Index Array(array=w509, index=0) -> (element=w518:u32)
        n307 = Index Array(array=w509, index=1) -> (element=w517:u32)
        n308 = Index Array(array=w509, index=2) -> (element=w516:u32)
        n309 = Index Array(array=w509, index=3) -> (element=w510:u32)
        n310 = Index Array(array=w509, index=4) -> (element=w511:u32)
        n311 = Index Array(array=w509, index=5) -> (element=w512:u32)
        n312 = Index Array(array=w509, index=6) -> (element=w513:u32)
        n313 = Index Array(array=w509, index=7) -> (element=w514:u32)
        n314 = Subtract(x=w518, y=w515) -> (x-y=→"单体温度16":u32)
        n315 = Subtract(x=w517, y=w515) -> (x-y=→"单体温度17":u32)
        n316 = Subtract(x=w516, y=w515) -> (x-y=→"单体温度18":u32)
        n317 = Subtract(x=w510, y=w515) -> (x-y=→"单体温度19":u32)
        n318 = Subtract(x=w511, y=w515) -> (x-y=→"单体温度20":u32)
        n319 = Subtract(x=w512, y=w515) -> (x-y=→"单体温度21":u32)
        n320 = Subtract(x=w513, y=w515) -> (x-y=→"单体温度22":u32)
        n321 = Subtract(x=w514, y=w515) -> (x-y=→"单体温度23":u32)
      }
      frame 408113395 {
        w541 = u8 40
        n322 = Index Array(array=w535, index=0) -> (element=w544:u32)
        n323 = Index Array(array=w535, index=1) -> (element=w543:u32)
        n324 = Index Array(array=w535, index=2) -> (element=w542:u32)
        n325 = Index Array(array=w535, index=3) -> (element=w536:u32)
        n326 = Index Array(array=w535, index=4) -> (element=w537:u32)
        n327 = Index Array(array=w535, index=5) -> (element=w538:u32)
        n328 = Index Array(array=w535, index=6) -> (element=w539:u32)
        n329 = Index Array(array=w535, index=7) -> (element=w540:u32)
        n330 = Subtract(x=w544, y=w541) -> (x-y=→"单体温度24":u32)
        n331 = Subtract(x=w543, y=w541) -> (x-y=→"单体温度25":u32)
        n332 = Subtract(x=w542, y=w541) -> (x-y=→"单体温度26":u32)
        n333 = Subtract(x=w536, y=w541) -> (x-y=→"单体温度27":u32)
        n334 = Subtract(x=w537, y=w541) -> (x-y=→"单体温度28":u32)
        n335 = Subtract(x=w538, y=w541) -> (x-y=→"单体温度29":u32)
        n336 = Subtract(x=w539, y=w541) -> (x-y=→"单体温度30":u32)
        n337 = Subtract(x=w540, y=w541) -> (x-y=→"单体温度31":u32)
      }
      frame 408178931 {
        w567 = u8 40
        n338 = Index Array(array=w561, index=0) -> (element=w570:u32)
        n339 = Index Array(array=w561, index=1) -> (element=w569:u32)
        n340 = Index Array(array=w561, index=2) -> (element=w568:u32)
        n341 = Index Array(array=w561, index=3) -> (element=w562:u32)
        n342 = Index Array(array=w561, index=4) -> (element=w563:u32)
        n343 = Index Array(array=w561, index=5) -> (element=w564:u32)
        n344 = Index Array(array=w561, index=6) -> (element=w565:u32)
        n345 = Index Array(array=w561, index=7) -> (element=w566:u32)
        n346 = Subtract(x=w570, y=w567) -> (x-y=→"单体温度32":u32)
        n347 = Subtract(x=w569, y=w567) -> (x-y=→"单体温度33":u32)
        n348 = Subtract(x=w568, y=w567) -> (x-y=→"单体温度34":u32)
        n349 = Subtract(x=w562, y=w567) -> (x-y=→"单体温度35":u32)
        n350 = Subtract(x=w563, y=w567) -> (x-y=→"单体温度36":u32)
        n351 = Subtract(x=w564, y=w567) -> (x-y=→"单体温度37":u32)
        n352 = Subtract(x=w565, y=w567) -> (x-y=→"单体温度38":u32)
        n353 = Subtract(x=w566, y=w567) -> (x-y=→"单体温度39":u32)
      }
      frame 408244467 {
        w593 = u8 40
        n354 = Index Array(array=w587, index=0) -> (element=w596:u32)
        n355 = Index Array(array=w587, index=1) -> (element=w595:u32)
        n356 = Index Array(array=w587, index=2) -> (element=w594:u32)
        n357 = Index Array(array=w587, index=3) -> (element=w588:u32)
        n358 = Index Array(array=w587, index=4) -> (element=w589:u32)
        n359 = Index Array(array=w587, index=5) -> (element=w590:u32)
        n360 = Index Array(array=w587, index=6) -> (element=w591:u32)
        n361 = Index Array(array=w587, index=7) -> (element=w592:u32)
        n362 = Subtract(x=w596, y=w593) -> (x-y=→"单体温度40":u32)
        n363 = Subtract(x=w595, y=w593) -> (x-y=→"单体温度41":u32)
        n364 = Subtract(x=w594, y=w593) -> (x-y=→"单体温度42":u32)
        n365 = Subtract(x=w588, y=w593) -> (x-y=→"单体温度43":u32)
        n366 = Subtract(x=w589, y=w593) -> (x-y=→"单体温度44":u32)
        n367 = Subtract(x=w590, y=w593) -> (x-y=→"单体温度45":u32)
        n368 = Subtract(x=w591, y=w593) -> (x-y=→"单体温度46":u32)
        n369 = Subtract(x=w592, y=w593) -> (x-y=→"单体温度47":u32)
      }
      frame 402780992 {
        w609 = u16 0
        n370 = Index Array(array=w610, index=0) -> (element=w606:u32)
        n371 = Index Array(array=w610, index=1) -> (element=w605:u32)
        n372 = Index Array(array=w610, index=2) -> ()  [unwired: 1 out]
        n373 = Index Array(array=w610, index=3) -> ()  [unwired: 1 out]
        n374 = Index Array(array=w610, index=4) -> ()  [unwired: 1 out]
        n375 = Index Array(array=w610, index=5) -> ()  [unwired: 1 out]
        n376 = Index Array(array=w610, index=6) -> ()  [unwired: 1 out]
        n377 = Index Array(array=w610, index=7) -> ()  [unwired: 1 out]
        n378 = Not Equal?(x=w609, y=w606) -> (x != y?=→"输出高压命令":bool)
        n379 = Not Equal?(x=w609, y=w605) -> (x != y?=→"关机命令":bool)
      }
      frame 34952 {
        n380 = Index Array(array=w620, index=0) -> (element=→"轮速":u32)
        n381 = Index Array(array=w620, index=1) -> ()  [unwired: 1 out]
        n382 = Index Array(array=w620, index=2) -> ()  [unwired: 1 out]
        n383 = Index Array(array=w620, index=3) -> ()  [unwired: 1 out]
        n384 = Index Array(array=w620, index=4) -> ()  [unwired: 1 out]
        n385 = Index Array(array=w620, index=5) -> ()  [unwired: 1 out]
        n386 = Index Array(array=w620, index=6) -> ()  [unwired: 1 out]
        n387 = Index Array(array=w620, index=7) -> ()  [unwired: 1 out]
      }
    }
  }
  n388 = VISA Close(VISA resource name=w4, error in (no error)=w3) -> ()  [unwired: 1 out]
